vi "PH_Sequencer.PC PPTimeoutSM.vi"(0 "i ref in":refnum<vi>, 2 "Power Unit":T2, 3 "SM Timeout":T1, 5 "error in (no error)":errorcluster) -> (14 "i ref out":refnum<vi>, 19 "error out":errorcluster)   [LabVIEW 2014, in "PH_Sequencer.lvlib"]
doc: "This VI writes the state of the timeout state machine of the related PU to own attributes."
uses:
  PH_Sequencer.lvlib
  PH_PP_Common/PH_PP_Common.PUs.ctl
  PH_PowerUnit_BaseClass/PH_PowerUnit_BaseClass.SM States.ctl
  PH_PowerUnit_BaseClass/PH_PowerUnit_BaseClass.lvlib
  PH_PP_Common/PH_PP_Common.lvlib
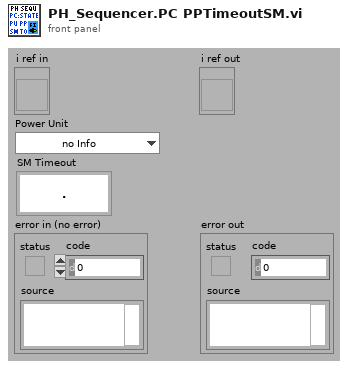
[diagram p1: front panel]
types:
  T1 = typedef "PH_PowerUnit_BaseClass.lvlib/PH_PowerUnit_BaseClass.SM States.ctl" = enum16{".", "Stand by", "Switch PU on", "Configure", "Set Default Voltage", "Set STANDBY", "Set READY", "Wait for Shot Cmd", "Open Dump Rods", "Open Ross Relais", "Close Ross Relais", "Switch PSU on", "Switch PSU off", "Charge", "Switch GD Channel on", "Close Dump Rods", "Rods-TO", "RR-TO", "PSU-TO", "Trigger-TO"}
  T2 = typedef "PH_PP_Common.lvlib/PH_PP_Common.PUs.ctl" = enum16{"no Info", "PA-19mm-1", "PA-19mm-2", "PA-45mm-PILC", "PA-45mm-MAIN", "MA-PU-1", "MA-PU-2", "MA-PU-3", "MA-PU-4", "MA-PU-5", "MA-PU-6", "MA-FR", "MA-PILC", "PA-45mm-DP"}
  T3 = typedef "PH_Sequencer.lvlib/PH_Sequencer.i attribute.ctl" = cluster{"GUI Refs":cluster{"Main Off":refnum<vi>, "Fire":refnum<vi>, "Status":refnum<vi>, "Ready":refnum<vi>, "Waiting Time":refnum<vi>, "Timeout":refnum<vi>, "PPMA Ready":refnum<vi>, "Sequencer SM State":refnum<vi>, "PPPA Ready":refnum<vi>, "Calorimeter":refnum<vi>, "Beamline Ready":refnum<vi>, "Clear Beamline":refnum<vi>, "Linkage PPMA Rods":refnum<vi>, "Linkage Current PA":refnum<vi>, "Linkage Current MA":refnum<vi>, "Timing Ready":refnum<vi>, "State Timing":refnum<vi>, "Force Timing":refnum<vi>, "PSDB Shot Comment":refnum<vi>, "State PA Backreflection":refnum<vi>, "Beamline Z6 Ready":refnum<vi>, "Clear Z6 Beamline":refnum<vi>, "Sequence length":refnum<vi>, "Timing Mode":refnum<vi>, "Slow Trigger Settings":refnum<vi>, "Experiment Description":refnum<vi>, "State PSDB":refnum<vi>, "PSDB Ready":refnum<vi>, "Set PSDB Settings":refnum<vi>, "Get PSDB Info":refnum<vi>, "Take Snapshot":refnum<vi>, "Shottype":refnum<vi>, "Experiment":refnum<vi>, "Phase Frontends":refnum<vi>, "PP 45mm PILC in use":refnum<vi>}, "Status Info":cluster{"Machine Status":T4, "WaitingTime":i32, "Timeout":bool}, "Readyness":cluster{"Ready to shot":bool, "PPMA Ready":bool, "PPPA Ready":bool, "BL Ready":bool, "Timing Ready":bool, "BL Z6 Ready":bool, "PSDBReady":bool}, "Instancenames":cluster{"PPMA Rods":string, "PP Current Meas":string, "PH Beamline Chief":string, "PA Backrefl Meas":string, "Z6 Beamline Chief":string}, "Data to read":bool, "Calorimeter":cluster{"Instancename":string, "On":bool, "linked":bool}, "Linkage":cluster{"PPMA Rods":bool, "PP Current Meas":bool, "PHELIX Beamline Chief":bool, "PA Backrefl Meas":bool, "Z6 Beamline Chief":bool}, "Timing":cluster{"Instance":string, "linked":bool, "Status":T4, "Timing Mode":T5, "Slow Trigger Settings":T6, "Info available":cluster{"ext SlowTrigger":bool, "T2":bool, "Mode":bool, "Delay Slow Trigger":bool, "Phase FEs":bool}, "FE Phase":T7}, "Service ID R2S":i32, "PSDB":cluster{"Controller Instance":string, "Controller Status":T4, "Controller linked":bool, "Settings acknowledged":bool, "Current Experiment ID":i16, "Current Shot Type":i16, "Current Comment":string, "Remember Settings":bool, "Write 2 early":bool}, "PSDB Data":cluster{"Main Off?":bool, "Sequence Length":dbl, "Sequence startet":timestamp}, "6P 4Q Positions":cluster{"Instancename":string, "linked":bool, "Position":T8}[], "PUs":T9[]}
  T4 = typedef "PH_StatusHandler.lvlib/PH_StatusHandler.Status.ctl" = i16
  T5 = typedef "PH_Timing.lvlib/PH_Timing.Timing Mode.ctl" = cluster{"T2":i16, "Modeselector":enum32{"10 Hz", "0.5 Hz", "Shot"}}
  T6 = typedef "PH_Timing.lvlib/PH_Timing.Slow Trigger Settings.ctl" = cluster{"Delay":dbl, "externally triggered?":bool}
  T7 = typedef "PH_Timing.lvlib/PH_Timing.Phase FEs.ctl" = cluster{"Phase":dbl}
  T8 = typedef "PH_4_Pos_Selector.lvlib/PH_4_Pos_Selector.Position Selector.ctl" = u16
  T9 = typedef "PH_Sequencer.lvlib/PH_Sequencer.Head.ctl" = cluster{"PowerUnit":T2, "GUI Ref":refnum<vi>, "Information":T10, "linked?":bool, "GUI Ref Current Voltage":refnum<vi>}
  T10 = typedef "PH_Sequencer.lvlib/PH_Sequencer.PU Information.ctl" = cluster{"State":T4, "Waiting Time [s]":dbl, "PU State SM":T1, "PU Timeout SM":T1}
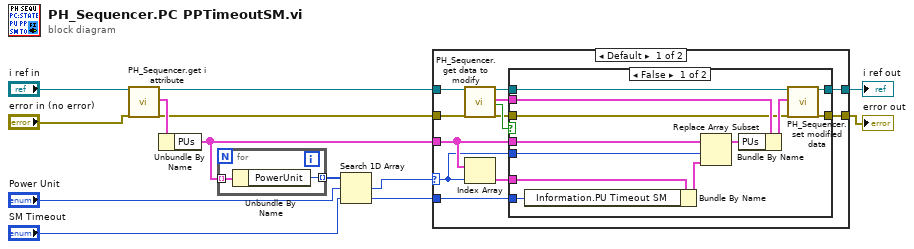
[diagram p0: block diagram]
diagram:
  n1 = call "PH_Sequencer.get i attribute.vi"("i ref in"="i ref in", "error in (no error)"="error in (no error)") -> ("i ref out"=w2:refnum<vi>, "i attribute"=w9:T3, "error out"=w4:errorcluster)  [unwired: 15 in]
  n2 = Unbundle By Name(w9) -> ("PUs"=w10:T9[])
  n3 = for {
    tunnel: w10 -> [w14] mode=indexing
    tunnel: [w13] -> w12 mode=indexing
    n4 = Unbundle By Name(w14) -> ("PowerUnit"=w13:T2)
  }
  n5 = Search 1D Array(1D array=w12, element="Power Unit") -> (index of element=w11:i32)  [unwired: 1 in]
  n6 = case shown="Default" w11 {
    selector: w11 -> [w24 _]
    tunnel: w10 -> [w26 _]
    tunnel: "SM Timeout" -> [w19 _]
    tunnel: [w18 w42] -> w6
    tunnel: [w17 w41] -> w7
    tunnel: w4 -> [w16 w41]
    tunnel: w2 -> [w15 w42]
    frame Default {
      n7 = call "PH_Sequencer.get data to modify.vi"("i ref in"=w15, "error in (no error)"=w16) -> ("i ref out"=w20:refnum<vi>, "i attribute"=w22:T3, "timed out"=w23:bool, "error out"=w21:errorcluster)  [unwired: 14 in]
      n8 = Index Array(array=w26, index=w24) -> (element=w25:T9)
      n9 = case shown="False" w23 {
        tunnel: w20 -> [w34 w40]
        tunnel: [w38 w40] -> w18
        tunnel: w21 -> [w27 w39]
        tunnel: [w37 w39] -> w17
        tunnel: w22 -> [w36 _]
        tunnel: w19 -> [w29 _]
        tunnel: w25 -> [w28 _]
        tunnel: w24 -> [w32 _]
        tunnel: w26 -> [w31 _]
        frame False {
          n10 = Bundle By Name(cluster=w28, "Information.PU Timeout SM"=w29) -> (w33:T9)
          n11 = Replace Array Subset(array=w31, new element=w33, index=w32) -> (w30:T9[])
          n12 = Bundle By Name(cluster=w36, "PUs"=w30) -> (w35:T3)
          n13 = call "PH_Sequencer.set modified data.vi"("i ref in"=w34, "i attribute"=w35, "error in (no error)"=w27) -> ("i ref out"=w38:refnum<vi>, "error out"=w37:errorcluster)  [unwired: 15 in]
        }
        frame True {
        }
      }
    }
    frame -1 {
    }
  }
  "error out" <- w7
  "i ref out" <- w6
